vi "Generate Mask.vi"(8 "error in (no error)":errorcluster, 10 "Parameter":string, 11 "1553 SubComponent in":refnum<class "1553 SubComponent.lvclass">) -> (0 "error out":errorcluster, 3 "1553 SubComponent out":refnum<class "1553 SubComponent.lvclass">)   [LabVIEW 2020, in "BCI-1553 API.lvlib" / "1553 SubComponent.lvclass"]
doc: "Automatically generates a mask for the parameter of interest. The parameter must already be in the write table."
uses:
  1553 SubComponent.lvclass
  Frames & Messages/TypeDefs/Parameter Table Data.ctl
  Frames & Messages/TypeDefs/Scaling Information.ctl
  1553 SubComponent.lvclass/1553 SubComponent.ctl
  Dependencies/Registry/Registry.lvclass/Registry.ctl
  Dependencies/Registry/Registry.lvclass
  BCI-1553 API.lvlib
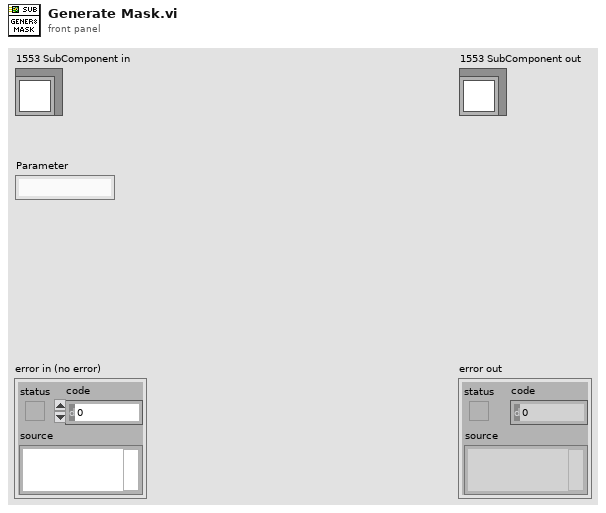
[diagram p1: front panel]
types:
  T1 = typedef "BCI-1553 API.lvlib/Parameter Table Data.ctl" = cluster{"Parameter Name":string, "Base Word":u16, "Address":u16, "Value":u64, "Mask":u16[], "Scaling Info":T2}
  T2 = typedef "BCI-1553 API.lvlib/Scaling Information.ctl" = cluster{"Bit Offset":i32, "Bit Count":i32, "LSB Resolution":dbl, "2's Complement":bool, "Big Endian":bool, "Sign Bit":bool}
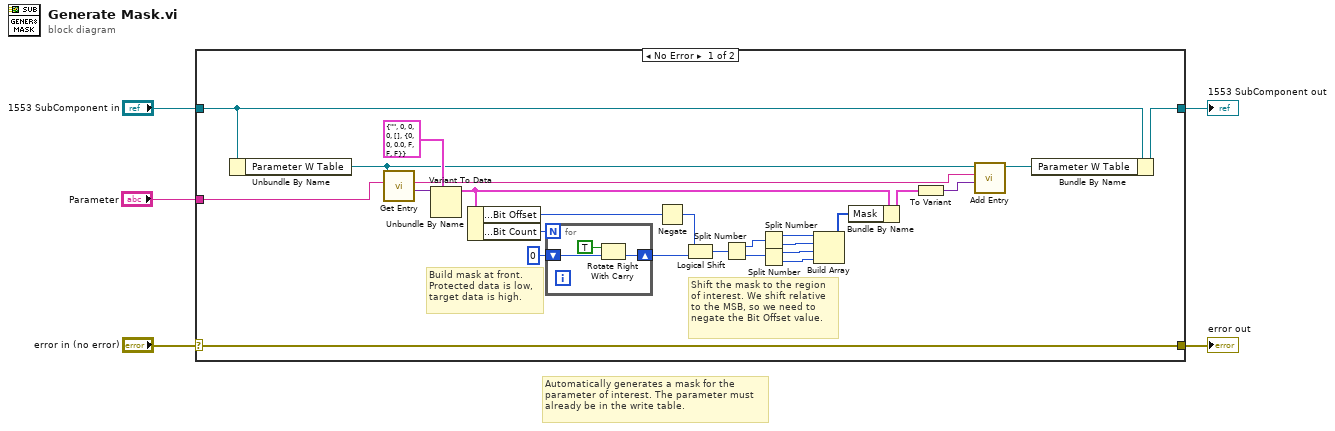
[diagram p0: block diagram]
diagram:
  # "Automatically generates a mask for the\nparameter of interest. The parameter must\nalready be in the write table."
  n1 = case shown="No Error" "error in (no error)" {
    selector: "error in (no error)" -> [w30 w35]
    tunnel: [w30 w35] -> w4
    tunnel: [w21 w34] -> w2
    tunnel: "1553 SubComponent in" -> [w22 w34]
    tunnel: "Parameter" -> [w19 _]
    frame No Error {
      # "Shift the mask to the region\nof interest. We shift relative\nto the MSB, so we need to\nnegate the Bit Offset value."
      # "Build mask at front.\nProtected data is low,\ntarget data is high."
      n2 = Unbundle By Name(w22) -> ("Parameter W Table"=w23:refnum<class "Registry.lvclass">)
      n3 = call "Get Entry.vi"("Key"=w19, "Registry in"=w23) -> ("Value"=w26:variant, "Key Out"=w24:string)  [unwired: 6 in, 2 out]
      n4 = Variant To Data(type=T1 {"Parameter Name"="", "Base Word"=0, "Address"=0, "Value"=0, "Mask"=[], "Scaling Info"={"Bit Offset"=0, "Bit Count"=0, "LSB Resolution"=0.0, "2's Complement"=FALSE, "Big Endian"=FALSE, "Sign Bit"=FALSE}} ("Parameter Table Data"), Variant=w26) -> (data=w28:T1)  [unwired: 1 in, 1 out]
      n5 = Unbundle By Name(w28) -> ("Scaling Info.Bit Offset"=w7:i32, "Scaling Info.Bit Count"=w18:i32)
      n6 = for {
        N: w18 -> [_]
        shift-right: [w32] -> w16
        shift-left: u64 0 -> [w33]
        n7 = Rotate Right With Carry(2:w33, 3:TRUE ("carry")) -> (0:w32:u64)  [unwired: 1 out]
      }
      n8 = Negate(x=w7) -> (-x=w6:i32)
      n9 = Logical Shift(y=w6, x=w16) -> (x << y=w9:u64)
      n10 = Split Number(x=w9) -> (hi(x)=w10:u32, lo(x)=w15:u32)
      n11 = Split Number(x=w10) -> (hi(x)=w14:u16, lo(x)=w13:u16)
      n12 = Split Number(x=w15) -> (hi(x)=w12:u16, lo(x)=w11:u16)
      n13 = Build Array(w14, w13, w12, w11) -> (w8:u16[])
      n14 = Bundle By Name(cluster=w28, "Mask"=w8) -> (w27:T1)
      n15 = To Variant(anything=w27) -> (Variant=w25:variant)
      n16 = call "Add Entry.vi"("Value"=w25, "Key"=w24, "Registry in"=w23) -> ("Registry out"=w20:refnum<class "Registry.lvclass">)  [unwired: 6 in, 2 out]
      n17 = Bundle By Name(cluster=w22, "Parameter W Table"=w20) -> (w21:refnum<class "1553 SubComponent.lvclass">)
    }
    frame Error {
    }
  }
  "error out" <- w4
  "1553 SubComponent out" <- w2
